vi "Classify Dependencies.vi"(0 "dependency paths":path[](array[path])) -> (4 "actual dependencies":path[](array[path]), 6 "driver vis":path[](array[path]))   [LabVIEW 2021, in "Multiple Converter.lvlib"]
uses:
  Multiple Converter.lvlib
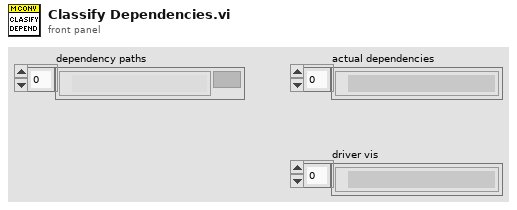
[diagram p1: front panel]
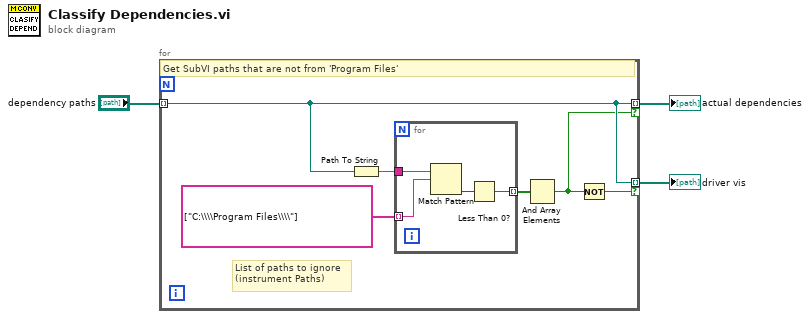
[diagram p0: block diagram]
diagram:
  n1 = for {
    tunnel: "dependency paths" -> [w8] mode=indexing
    tunnel: [w8] -> w3 mode=indexing if=w4
    tunnel: [w8] -> w1 mode=indexing if=w5
    # "List of paths to ignore\n(instrument Paths)"
    # "Get SubVI paths that are not from 'Program Files'"
    n2 = Path To String(path=w8) -> (string=w9:string)
    n3 = for {
      tunnel: w9 -> [w13]
      tunnel: [w11] -> w7 mode=indexing
      tunnel: string[] ["C:\\\\Program Files\\\\"] -> [w10] mode=indexing
      n4 = Match Pattern(string=w13, regular expression=w10) -> (offset past match=w12:i32)  [unwired: 1 in, 3 out]
      n5 = Less Than 0?(x=w12) -> (x < 0?=w11:bool)
    }
    n6 = And Array Elements(Boolean array=w7) -> (logical AND=w4:bool)
    n7 = Not(x=w4) -> (.not. x?=w5:bool)
  }
  "actual dependencies" <- w3
  "driver vis" <- w1
